vi "get_pid_configuration.vi"(8 "error in (no error)":errorcluster, 11 "VISA Refnum in":refnum<visa-resource-name>) -> (0 "error out":errorcluster, 1 "Disable adaptive control":bool, 2 "Control action":string, 3 "VISA Refnum out":refnum<visa-resource-name>)   [LabVIEW 2018]
panel:
  in  "Control actions":string(combo)="0"
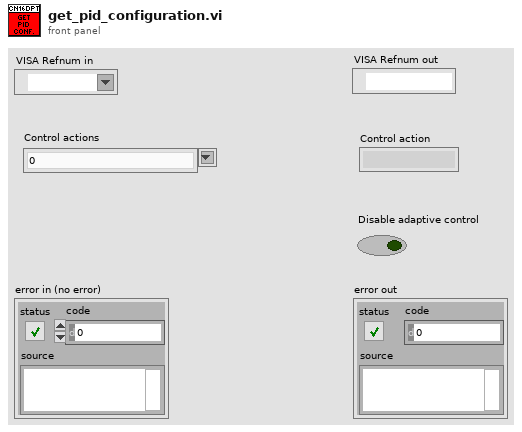
[diagram p1: front panel]
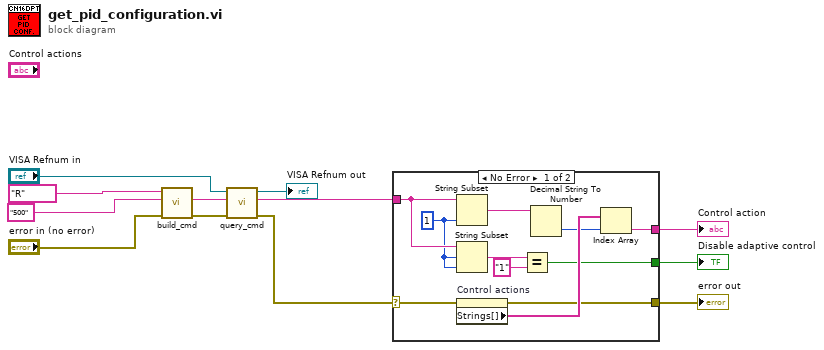
[diagram p0: block diagram]
diagram:
  n1 = call "build_cmd.vi"("error in (no error)"="error in (no error)", "Command ID"="500", "Command class"="R") -> ("error out"=w7:errorcluster, "Command"=w6:string)  [unwired: 7 in]
  n2 = call "query_cmd.vi"("error in (no error)"=w7, "Command"=w6, "VISA resource name"="VISA Refnum in") -> ("error out"=w2:errorcluster, "Response"=w5:string, "VISA resource name out"=→"VISA Refnum out":refnum<visa-resource-name>)  [unwired: 6 in]
  n3 = case shown="No Error" w2 {
    selector: w2 -> [w14 w24]
    tunnel: w5 -> [w23 _]
    tunnel: [w18 _] -> w4
    tunnel: [w15 _] -> w3
    tunnel: [w13 w24] -> w1
    frame No Error {
      w21 = 1 ("length (rest)")
      n4 = String Subset(string=w23, length (rest)=w21) -> (substring=w20:string)  [unwired: 1 in]
      n5 = String Subset(string=w23, offset (0)=w21, length (rest)=w21) -> (substring=w17:string)
      n6 = property on="Control actions" class="CmbBox"(error in=w14) -> (error out=w13:errorcluster, "Strings[]"=w22:string[])  [unwired: 1 in, 1 out]
      n7 = Equal?(x=w17, y="1") -> (x = y?=w15:bool)
      n8 = Decimal String To Number(string=w20) -> (number=w19:i32)  [unwired: 2 in, 1 out]
      n9 = Index Array(array=w22, index=w19) -> (element=w18:string)
    }
    frame Error {
    }
  }
  "error out" <- w1
  "Disable adaptive control" <- w3
  "Control action" <- w4
